vi "USBTC08Example.vi"() -> ()   [LabVIEW 2017]
uses:
  Instance           1 15Saved   usbtc08 .vi
  Pico Temperature.vi
  usbtc08.dll
panel:
  in  "Mains Frequency":i16(ring) items=["50 Hz", "60 Hz"]
  out "?":dynamicdata(graph)
  in  "?":bool
  in  "Ch # 8":bool
  in  "Type # 8":i16(ring)=107 items=["B"=98, "E"=101, "J"=106, "K"=107, "N"=110, "R"=114, "S"=115, "T"=116, "Voltage"=120]
  in  "Ch # 7":bool
  in  "Type # 7":i16(ring)=107 items=["B"=98, "E"=101, "J"=106, "K"=107, "N"=110, "R"=114, "S"=115, "T"=116, "Voltage"=120]
  in  "Ch # 6":bool
  in  "Type # 6":i16(ring)=107 items=["B"=98, "E"=101, "J"=106, "K"=107, "N"=110, "R"=114, "S"=115, "T"=116, "Voltage"=120]
  in  "Ch # 5":bool
  in  "Type # 5":i16(ring)=107 items=["B"=98, "E"=101, "J"=106, "K"=107, "N"=110, "R"=114, "S"=115, "T"=116, "Voltage"=120]
  in  "Ch # 4":bool
  in  "Type # 4":i16(ring)=107 items=["B"=98, "E"=101, "J"=106, "K"=107, "N"=110, "R"=114, "S"=115, "T"=116, "Voltage"=120]
  in  "Ch # 3":bool
  in  "Type # 3":i16(ring)=107 items=["B"=98, "E"=101, "J"=106, "K"=107, "N"=110, "R"=114, "S"=115, "T"=116, "Voltage"=120]
  in  "Ch# 2":bool=TRUE
  in  "Type # 2":i16(ring)=107 items=["B"=98, "E"=101, "J"=106, "K"=107, "N"=110, "R"=114, "S"=115, "T"=116, "Voltage"=120]
  in  "Ch# 1":bool=TRUE
  in  "Type # 1":i16(ring)=107 items=["B"=98, "E"=101, "J"=106, "K"=107, "N"=110, "R"=114, "S"=115, "T"=116, "Voltage"=120]
  in  "Units":enum16{"C°", "F°", "K°", "R°"}(ring)
  in  "stop":bool
  out "Handle":i16
  # "Display updated every 2 seconds"
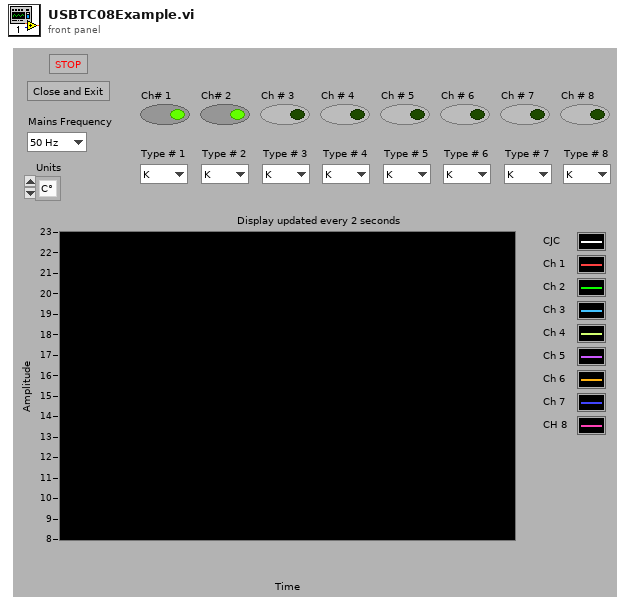
[diagram p1: front panel]
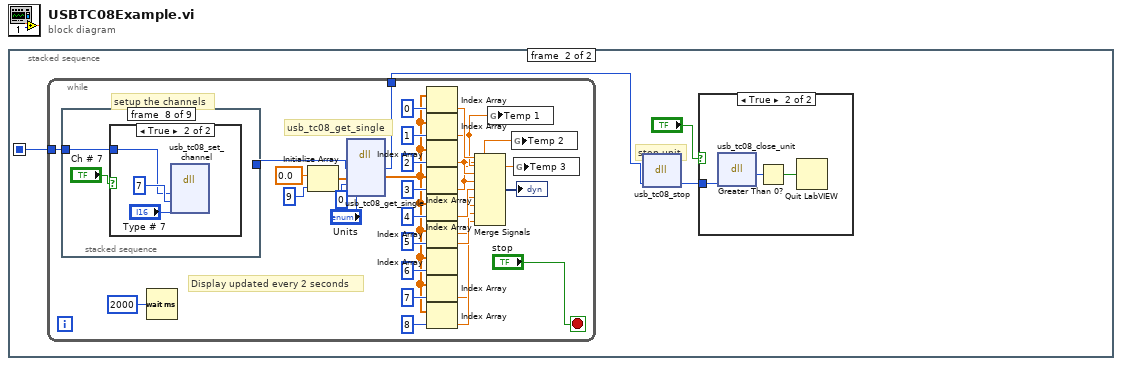
[diagram p0: block diagram]
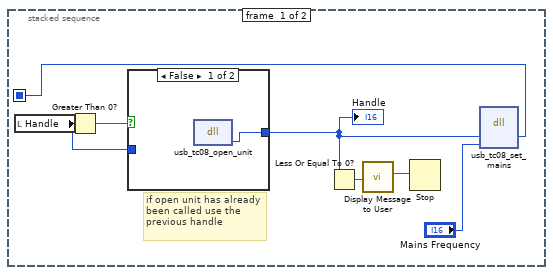
[diagram p2: hidden frame]
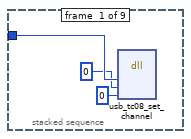
[diagram p4: hidden frame]
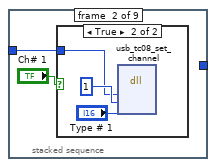
[diagram p5: hidden frame]
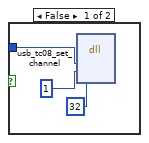
[diagram p6: hidden frame]
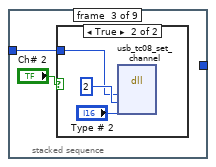
[diagram p7: hidden frame]
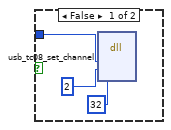
[diagram p8: hidden frame]
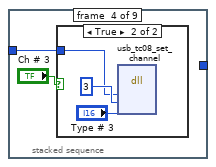
[diagram p9: hidden frame]
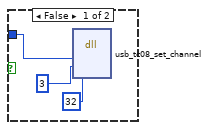
[diagram p10: hidden frame]
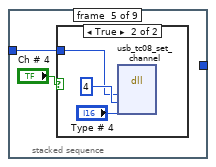
[diagram p11: hidden frame]
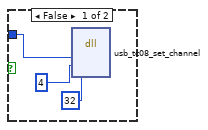
[diagram p12: hidden frame]
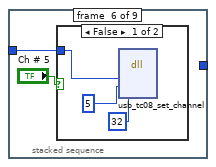
[diagram p13: hidden frame]
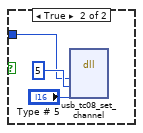
[diagram p14: hidden frame]
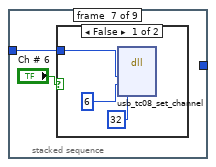
[diagram p15: hidden frame]
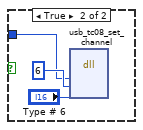
[diagram p16: hidden frame]
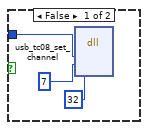
[diagram p17: hidden frame]
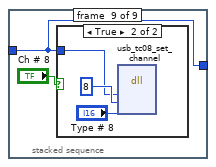
[diagram p18: hidden frame]
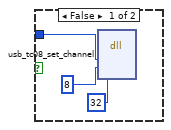
[diagram p19: hidden frame]
diagram:
  n1 = stacked-sequence {
    seq-local: [w5 _] -> [_ w13]
    frame #0 {
      # "if open unit has already been called use the previous handle"
      n2 = local read "Handle"() -> (w6:i16)
      n3 = Greater Than 0?(x=w6) -> (x > 0?=w7:bool)
      n4 = case shown="False" w7 {
        tunnel: [w8 w9] -> w4
        tunnel: w6 -> [_ w9]
        frame False {
          n5 = dll-call lib="usbtc08.dll" fn="usb_tc08_open_unit" label="OpenUnit"() -> ("Handle"=w8:i16)  [unwired: 3 in, 2 out]
        }
        frame True {
        }
      }
      "Handle" <- w4
      n6 = Less Or Equal To 0?(x=w4) -> (x <= 0?=w3:bool)
      n7 = call "Display Message to User"("Enable"=w3) -> ("OK"=w2:bool)  [unwired: 9 in, 1 out]
      n8 = Stop(stop? (T)=w2) -> ()
      n9 = dll-call lib="usbtc08.dll" fn="usb_tc08_set_mains" label="Set Mains"("Handle"=w4, "sixtyHertz"="Mains Frequency") -> ("Handle"=w5:i16)  [unwired: 5 in, 2 out]
    }
    frame #1 {
      # "stop unit"
      n10 = while {
        tunnel: w13 -> [w43]
        tunnel: [w19] -> w10
        stop <- "stop" stop-if-true
        # "Display updated every 2 seconds"
        # "usb_tc08_get_single"
        # "setup the channels"
        n11 = stacked-sequence {
          tunnel: w43 -> [w46 w48 w56 w64 w72 w80 w88 w96 w103]
          tunnel: [_ _ _ _ _ _ _ _ w103] -> w39
          frame #0 {
            n12 = dll-call lib="usbtc08.dll" fn="usb_tc08_set_channel"("handle"=w46, "channel"=i16 0, "tc_type"=i8 0) -> ()  [unwired: 7 in, 2 out]
          }
          frame #1 {
            n13 = case shown="True" "Ch# 1" {
              tunnel: w48 -> [w50 w53]
              frame False {
                n14 = dll-call lib="usbtc08.dll" fn="usb_tc08_set_channel"("handle"=w50, "channel"=i16 1, "tc_type"=32) -> ()  [unwired: 7 in, 2 out]
              }
              frame True {
                n15 = dll-call lib="usbtc08.dll" fn="usb_tc08_set_channel"("handle"=w53, "channel"=i16 1, "tc_type"="Type # 1") -> ()  [unwired: 7 in, 2 out]
              }
            }
          }
          frame #2 {
            n16 = case shown="True" "Ch# 2" {
              tunnel: w56 -> [w57 w61]
              frame False {
                n17 = dll-call lib="usbtc08.dll" fn="usb_tc08_set_channel"("handle"=w57, "channel"=i16 2, "tc_type"=32) -> ()  [unwired: 7 in, 2 out]
              }
              frame True {
                n18 = dll-call lib="usbtc08.dll" fn="usb_tc08_set_channel"("handle"=w61, "channel"=i16 2, "tc_type"="Type # 2") -> ()  [unwired: 7 in, 2 out]
              }
            }
          }
          frame #3 {
            n19 = case shown="True" "Ch # 3" {
              tunnel: w64 -> [w65 w69]
              frame False {
                n20 = dll-call lib="usbtc08.dll" fn="usb_tc08_set_channel"("handle"=w65, "channel"=i16 3, "tc_type"=32) -> ()  [unwired: 7 in, 2 out]
              }
              frame True {
                n21 = dll-call lib="usbtc08.dll" fn="usb_tc08_set_channel"("handle"=w69, "channel"=i16 3, "tc_type"="Type # 3") -> ()  [unwired: 7 in, 2 out]
              }
            }
          }
          frame #4 {
            n22 = case shown="True" "Ch # 4" {
              tunnel: w72 -> [w73 w77]
              frame False {
                n23 = dll-call lib="usbtc08.dll" fn="usb_tc08_set_channel"("handle"=w73, "channel"=i16 4, "tc_type"=32) -> ()  [unwired: 7 in, 2 out]
              }
              frame True {
                n24 = dll-call lib="usbtc08.dll" fn="usb_tc08_set_channel"("handle"=w77, "channel"=i16 4, "tc_type"="Type # 4") -> ()  [unwired: 7 in, 2 out]
              }
            }
          }
          frame #5 {
            n25 = case shown="False" "Ch # 5" {
              tunnel: w80 -> [w81 w85]
              frame False {
                n26 = dll-call lib="usbtc08.dll" fn="usb_tc08_set_channel"("handle"=w81, "channel"=i16 5, "tc_type"=32) -> ()  [unwired: 7 in, 2 out]
              }
              frame True {
                n27 = dll-call lib="usbtc08.dll" fn="usb_tc08_set_channel"("handle"=w85, "channel"=i16 5, "tc_type"="Type # 5") -> ()  [unwired: 7 in, 2 out]
              }
            }
          }
          frame #6 {
            n28 = case shown="False" "Ch # 6" {
              tunnel: w88 -> [w89 w93]
              frame False {
                n29 = dll-call lib="usbtc08.dll" fn="usb_tc08_set_channel"("handle"=w89, "channel"=i16 6, "tc_type"=32) -> ()  [unwired: 7 in, 2 out]
              }
              frame True {
                n30 = dll-call lib="usbtc08.dll" fn="usb_tc08_set_channel"("handle"=w93, "channel"=i16 6, "tc_type"="Type # 6") -> ()  [unwired: 7 in, 2 out]
              }
            }
          }
          frame #7 {
            n31 = case shown="True" "Ch # 7" {
              tunnel: w96 -> [w97 w101]
              frame False {
                n32 = dll-call lib="usbtc08.dll" fn="usb_tc08_set_channel"("handle"=w97, "channel"=i16 7, "tc_type"=32) -> ()  [unwired: 7 in, 2 out]
              }
              frame True {
                n33 = dll-call lib="usbtc08.dll" fn="usb_tc08_set_channel"("handle"=w101, "channel"=i16 7, "tc_type"="Type # 7") -> ()  [unwired: 7 in, 2 out]
              }
            }
          }
          frame #8 {
            n34 = case shown="True" "Ch # 8" {
              tunnel: w103 -> [w105 w109]
              frame False {
                n35 = dll-call lib="usbtc08.dll" fn="usb_tc08_set_channel"("handle"=w105, "channel"=i16 8, "tc_type"=32) -> ()  [unwired: 7 in, 2 out]
              }
              frame True {
                n36 = dll-call lib="usbtc08.dll" fn="usb_tc08_set_channel"("handle"=w109, "channel"=i16 8, "tc_type"="Type # 8") -> ()  [unwired: 7 in, 2 out]
              }
            }
          }
        }
        n37 = Wait (ms)(milliseconds to wait=u32 2000) -> ()  [unwired: 1 out]
        n38 = Initialize Array(sgl 0.0, i16 9) -> (w42:sgl[])
        n39 = dll-call lib="usbtc08.dll" fn="usb_tc08_get_single"("handle"=w39, "temp_buffer"=w42, "overflow"=i16 0, "units"="Units") -> ("handle"=w19:i16, "temp_buffer"=w27:sgl[])  [unwired: 6 in, 2 out]
        n40 = Index Array(array=w27, index=i16 0) -> (element=w26:sgl)
        n41 = Index Array(array=w27, index=i16 1) -> (element=w16:sgl)
        n42 = Index Array(array=w27, index=i16 2) -> (element=w15:sgl)
        n43 = Index Array(array=w27, index=i16 3) -> (element=w14:sgl)
        n44 = Index Array(array=w27, index=4) -> (element=w25:sgl)
        n45 = Index Array(array=w27, index=i16 5) -> (element=w24:sgl)
        n46 = Index Array(array=w27, index=6) -> (element=w23:sgl)
        n47 = Index Array(array=w27, index=i16 7) -> (element=w21:sgl)
        n48 = Index Array(array=w27, index=i16 8) -> (element=w22:sgl)
        n49 = Merge Signals(w26, w16, w15, w14, w25, w24, w23, w21, w22) -> (→"?":dynamicdata)
        n50 = global write "Pico Temperature.vi" "Temp 1"(w16) -> ()
        n51 = global write "Pico Temperature.vi" "Temp 2"(w15) -> ()
        n52 = global write "Pico Temperature.vi" "Temp 3"(w14) -> ()
      }
      n53 = dll-call lib="usbtc08.dll" fn="usb_tc08_stop" ("Close unit")("handle"=w10) -> ("handle"=w12:i16)  [unwired: 4 in, 2 out]
      n54 = case shown="True" "?" {
        tunnel: w12 -> [_ w113]
        frame False {
        }
        frame True {
          n55 = dll-call lib="usbtc08.dll" fn="usb_tc08_close_unit" ("Close unit")("handle"=w113) -> ("return type"=w112:i16)  [unwired: 4 in, 2 out]
          n56 = Greater Than 0?(x=w112) -> (x > 0?=w111:bool)
          n57 = Quit LabVIEW(quit? (T)=w111) -> ()
        }
      }
    }
  }
